vi "HW_6p1_Task1_fishele.vi"() -> ()   [LabVIEW 2021]
uses:
  <vilib>/express/express arith-compare/Formula/XNode/ExpressFormulaBlockNode.xnode
panel:
  out "Minutes":i32
  in  "Target Concentration of C (mol/L)":dbl=105.0
  out "Concentration of C (mol/L)":dbl
  out "Concentration of B (mol/L)":dbl
  out "Concentration of A (mol/L)":dbl
  in  "K3 (L^4/(mol^4*min)":dbl=9.6e-13
  in  "K2 (L/(mol*min)":dbl=3.44e-07
  in  "K1 (L^2/(mol^2*min)":dbl=4.6e-05
  in  "Initial Concentration B (mol/L)":dbl=330.0
  in  "Inital Concentration A (mol/L)":dbl=210.0
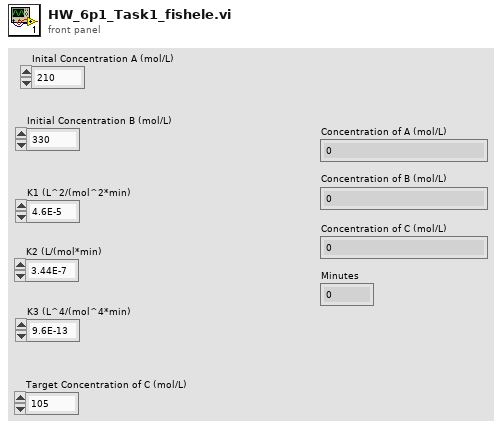
[diagram p1: front panel]
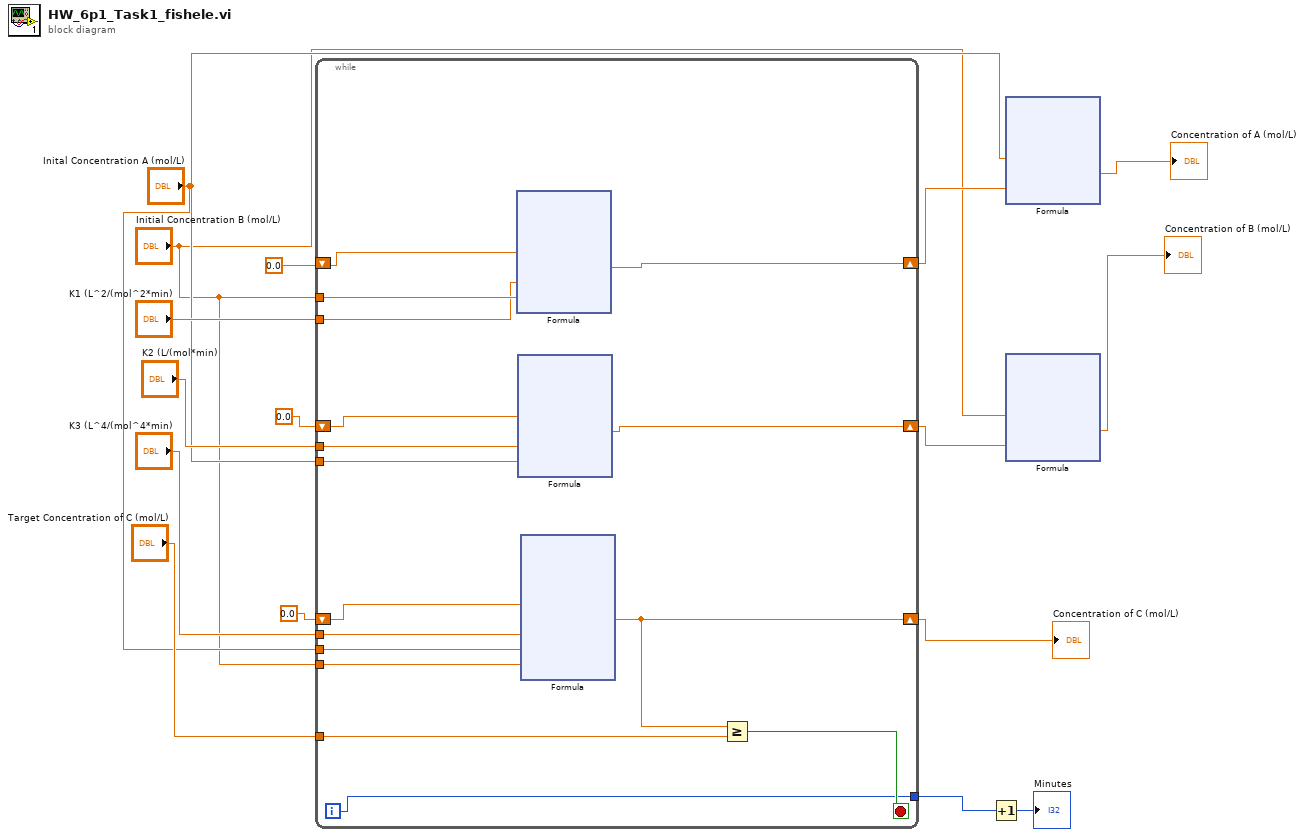
[diagram p0: block diagram]
diagram:
  n1 = while {
    shift-right: [w31] -> w6
    shift-left: 0.0 -> [w32]
    tunnel: "Initial Concentration B (mol/L)" -> [w30]
    tunnel: "K1 (L^2/(mol^2*min)" -> [w29]
    tunnel: "K2 (L/(mol*min)" -> [w28]
    tunnel: "Inital Concentration A (mol/L)" -> [w27]
    shift-right: [w26] -> w3
    shift-left: 0.0 ("Bconc") -> [w25]
    shift-right: [w19] -> w9
    shift-left: 0.0 ("Cconc") -> [w24]
    tunnel: "K3 (L^4/(mol^4*min)" -> [w23]
    tunnel: "Inital Concentration A (mol/L)" -> [w22]
    tunnel: "Initial Concentration B (mol/L)" -> [w21]
    tunnel: "Target Concentration of C (mol/L)" -> [w20]
    tunnel: [w17] -> w8
    i -> [w17]
    stop <- w18 stop-if-true
    n2 = xnode "Formula"("Aconc"=w32, "k1"=w29, "Bc"=w30) -> ("Result"=w31:dbl)  [unwired: 1 in, 1 out]
    n3 = xnode "Formula"("Bconc"=w25, "k2"=w28, "Ac"=w27) -> ("Result"=w26:dbl)  [unwired: 1 in, 1 out]
    n4 = xnode "Formula"("Cconc"=w24, "k3"=w23, "Ac"=w22, "Bc"=w21) -> ("Result"=w19:dbl)  [unwired: 1 in, 1 out]
    n5 = Greater Or Equal?(x=w19, y=w20) -> (x >= y?=w18:bool)
  }
  "Concentration of C (mol/L)" <- w9
  n6 = Increment(x=w8) -> (x+1=→"Minutes":i32)
  n7 = xnode "Formula"("Ac"="Inital Concentration A (mol/L)", "Aconc"=w6) -> ("Result"=→"Concentration of A (mol/L)":dbl)  [unwired: 1 in, 1 out]
  n8 = xnode "Formula"("Bc"="Initial Concentration B (mol/L)", "Bconc"=w3) -> ("Result"=→"Concentration of B (mol/L)":dbl)  [unwired: 1 in, 1 out]
